vi "Clip Plane of Scene.vi"() -> ()   [LabVIEW 2023]
doc: "This VI demonstrates how to use the clip plane in a 3D Picture and how to apply texture to objects, making them appear more realistic."
uses:
  <vilib>/Utility/miscctls.llb/LVPlaneTypeDef.ctl
  <vilib>/picture/3D Picture Control/Object/Create Object (name).vi
  <vilib>/picture/3D Picture Control/Object/Create Object (drawable).vi
  <vilib>/picture/3D Picture Control/Helpers/Apply Texture (no reference).vi
  <vilib>/picture/3D Picture Control/Object/Add Object (no reference).vi
  <vilib>/picture/3D Picture Control/Helpers/Set Clip Plane (reference).vi
  <vilib>/picture/3D Picture Control/NI_3D Picture Control.lvlib
panel:
  in  "Plane":T1 {"A" scale=-10.0..10.0; "B" scale=-10.0..10.0; "C" scale=-10.0..10.0; "D" scale=-100.0..100.0}
  out "3D Picture":refnum<vi>(3d-picture)
  in  "Stop":bool
  # "Overview: This VI demonstrates how to use the clip plane in a 3D Picture and how to apply texture to objects, making them appear more realistic. \nRequirements: LabVIEW Full Development System\nInstructions: \n1. Run the VI. \n2. Change Plane parameters and verify how the plane created by the equation A.X + B.Y + C.Z +D cuts the scene in that plane.\n3. Click Stop to stop the VI."
  # "Plane = A.x +B.y +C.z +D"
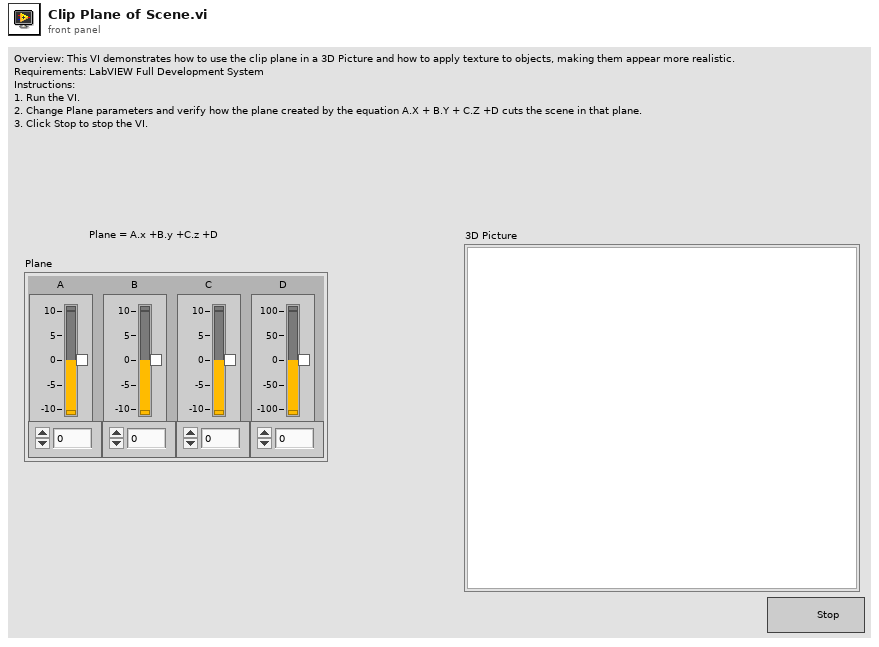
[diagram p1: front panel]
types:
  T1 = typedef "LVPlaneTypeDef.ctl" = cluster{"A":sgl, "B":sgl, "C":sgl, "D":sgl}
  T2 = enum16{"Inherit Value", "Points", "Wireframe", "Polygons"}
  T3 = enum16{"Inherit Value", "No Culling", "Cull Back Face", "Cull Front Face", "Cull Both Faces"}
  T4 = typedef "imagedata.ctl" = cluster{"image type":i32, "image depth":i32, "image":u8[], "mask":u8[], "colors":u32[], "Rectangle":cluster{"left":i16, "top":i16, "right":i16, "bottom":i16}}
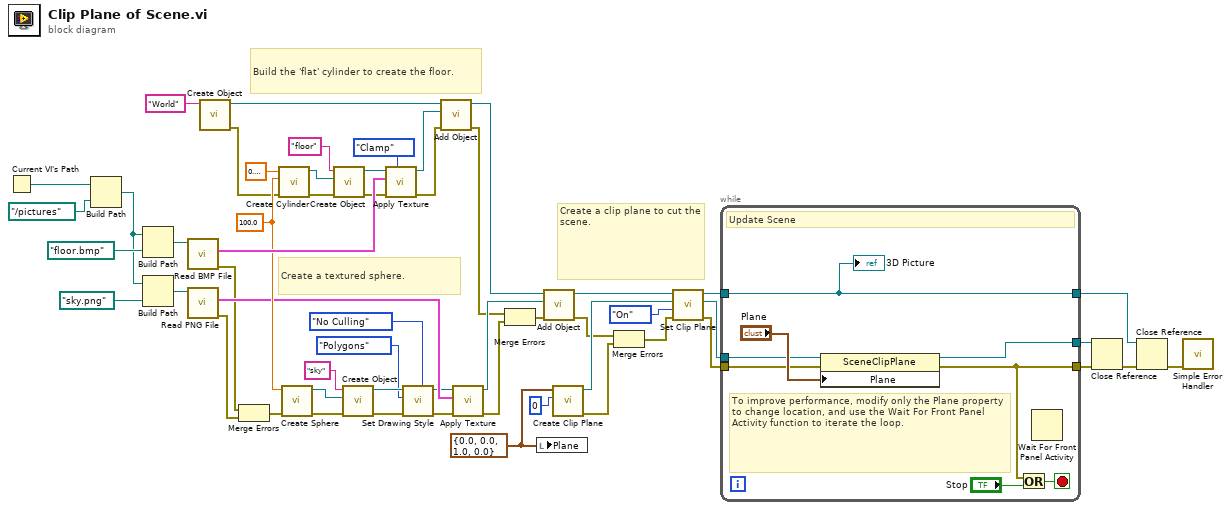
[diagram p0: block diagram]
diagram:
  w12 = cluster{"A":sgl, "B":sgl, "C":sgl, "D":sgl} {"A"=0.0, "B"=0.0, "C"=1.0, "D"=0.0} ("Plane")
  w46 = sgl 100.0 ("Height")
  # "Create a textured sphere."
  # "Create a clip plane to cut the scene."
  # "Build the 'flat' cylinder to create the floor."
  n1 = Current VI's Path() -> (path=w7:path)
  n2 = Build Path(base path=w7, name or relative path=path "../pictures" ("stripped path")) -> (appended path=w29:path)
  n3 = Build Path(base path=w29, name or relative path=path "floor.bmp") -> (appended path=w55:path)
  n4 = Build Path(base path=w29, name or relative path=path "sky.png") -> (appended path=w28:path)
  n5 = call <vilib>:"Read BMP File.vi"("path to BMP file"=w55) -> ("error out"=w10:errorcluster, "image data"=w54:T4)  [unwired: 8 in, 1 out]
  n6 = call <vilib>:"Read PNG File.vi"("path to PNG file"=w28) -> ("error out"=w9:errorcluster, "image data"=w35:T4)  [unwired: 8 in, 1 out]
  n7 = call-poly <vilib>:"Create Object.vi"("Name"="World") -> ("error out"=w11:errorcluster, "Scene:New Object"=w15:refnum<vi>)  [unwired: 9 in]
  n8 = Merge Errors(w10, w9) -> (w8:errorcluster)
  n9 = call <vilib>:"Create Cylinder.vi"("error in (no error)"=w11, "Radius"=w46, "Height"=sgl 0.1) -> ("error out"=w45:errorcluster, "New Cylinder Refnum"=w52:refnum<vi>)  [unwired: 7 in]
  n10 = call <vilib>:"Create Sphere.vi"("error in (no error)"=w8, "Radius"=w46) -> ("error out"=w42:errorcluster, "New Sphere Refnum"=w41:refnum<vi>)  [unwired: 8 in]
  n11 = call-poly <vilib>:"Create Object.vi"("error in (no error)"=w45, "Geometry"=w52, "Name"="floor") -> ("error out"=w44:errorcluster, "Scene:New Object"=w50:refnum<vi>)  [unwired: 7 in]
  n12 = call-poly <vilib>:"Create Object.vi"("error in (no error)"=w42, "Geometry"=w41, "Name"="sky") -> ("error out"=w40:errorcluster, "Scene:New Object"=w39:refnum<vi>)  [unwired: 7 in]
  n13 = call-poly <vilib>:"Apply Texture.vi"("Horizontal Wrap Mode"=enum16{"Clamp", "Repeat"}."Clamp", "error in (no error)"=w44, "Image Data"=w54, "Scene Object In"=w50) -> ("error out"=w43:errorcluster, "Scene Object Out"=w49:refnum<vi>)  [unwired: 6 in]
  n14 = call <vilib>:"Set Drawing Style.vi"("Face Culling Mode"=T3."No Culling" ("Draw Style:Face Culling Mode"), "error in (no error)"=w40, "Mode"=T2."Polygons" ("Draw Style:Mode"), "Scene Object In"=w39) -> ("error out"=w27:errorcluster, "Scene Object Out"=w34:refnum<vi>)  [unwired: 6 in]
  n15 = call-poly <vilib>:"Add Object.vi"("error in (no error)"=w43, "New Object In"=w49, "Scene Object In"=w15) -> ("error out"=w23:errorcluster, "Scene Object Out"=w26:refnum<vi>)  [unwired: 7 in]
  n16 = call-poly <vilib>:"Apply Texture.vi"("error in (no error)"=w27, "Image Data"=w35, "Scene Object In"=w34) -> ("error out"=w24:errorcluster, "Scene Object Out"=w25:refnum<vi>)  [unwired: 7 in]
  n17 = Merge Errors(w23, w24) -> (w22:errorcluster)
  n18 = local write "Plane"(w12) -> ()
  n19 = call-poly <vilib>:"Add Object.vi"("error in (no error)"=w22, "New Object In"=w25, "Scene Object In"=w26) -> ("error out"=w18:errorcluster, "Scene Object Out"=w17:refnum<vi>)  [unwired: 7 in]
  n20 = call <vilib>:"Create Clip Plane.vi"("Number"=0, "Plane"=w12) -> ("error out"=w21:errorcluster, "New Clip Plane Refnum"=w32:refnum<vi>)  [unwired: 8 in]
  n21 = Merge Errors(w18, w21) -> (w16:errorcluster)
  n22 = call-poly <vilib>:"Set Clip Plane.vi"("error in (no error)"=w16, "Clip Plane State"=enum16{"Inherit Value", "Off", "On"}."On", "Clip Plane Refnum In"=w32, "Scene Object In"=w17) -> ("error out"=w13:errorcluster, "Clip Plane Refnum Out"=w4:refnum<vi>, "Scene Object Out"=w14:refnum<vi>)  [unwired: 5 in]
  n23 = while {
    tunnel: w14 -> [w57]
    tunnel: w4 -> [w61]
    tunnel: w13 -> [w60]
    tunnel: [w58] -> w2
    tunnel: [w57] -> w6
    tunnel: [w56] -> w1
    stop <- w59 stop-if-true
    # "To improve performance, modify only the Plane property to change location, and use the Wait For Front Panel Activity function to iterate the loop."
    # "Update Scene"
    n24 = property class="SceneClipPlane"(reference=w61, error in=w60, "Plane"="Plane") -> (reference out=w56:refnum<vi>, error out=w58:errorcluster)
    n25 = Or(x=w58, y="Stop") -> (x .or. y?=w59:bool)
    n26 = Wait For Front Panel Activity() -> ()  [unwired: 3 in, 1 out]
    "3D Picture" <- w57
  }
  n27 = Close Reference(reference=w1, error in (no error)=w2) -> (error out=w3:errorcluster)
  n28 = Close Reference(reference=w6, error in (no error)=w3) -> (error out=w5:errorcluster)
  n29 = call <vilib>:"Simple Error Handler.vi"("error in (no error)"=w5) -> ()  [unwired: 4 in, 5 out]
